vi "SSH_Session.vi"(9 "Processor":i32=2, 11 "Python version":string="3.7") -> (0 "error out":errorcluster, 3 "Python":T1)   [LabVIEW 2019]
uses:
  SerialVIs/PythonCtrl.ctl
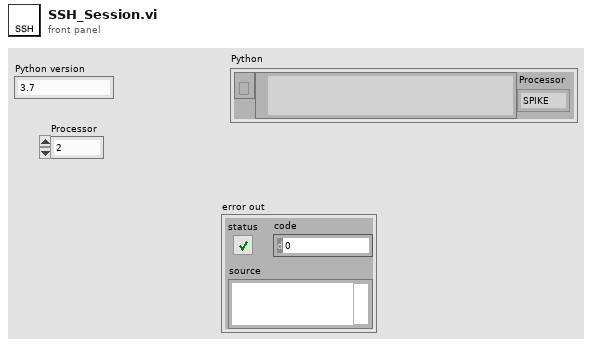
[diagram p1: front panel]
types:
  T1 = typedef "PythonCtrl.ctl" = cluster{"session":refnum<k35>, "PyPath":path, "Processor":enum16{"SPIKE", "Pi", "Pi_ssh"}}
  T2 = cluster{"session out":refnum<k35>, "appended path":path, "Processor":i32}
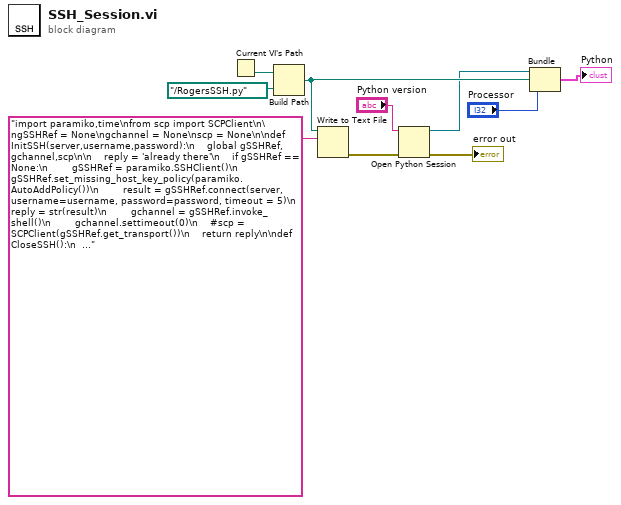
[diagram p0: block diagram]
diagram:
  n1 = Current VI's Path() -> (path=w5:path)
  n2 = Build Path(base path=w5, name or relative path=path "../RogersSSH.py" ("base path")) -> (appended path=w7:path)
  n3 = Write to Text File(file (use dialog)=w7, text="import paramiko,time\nfrom scp import SCPClient\n\ngSSHRef = None\ngchannel = None\nscp = None\n\ndef InitSSH(server,username,password):\n    global gSSHRef, gchannel,scp\n\n    reply = 'already there'\n    if gSSHRef == None:\n        gSSHRef = paramiko.SSHClient()\n        gSSHRef.set_missing_host_key_policy(paramiko.AutoAddPolicy())\n        result = gSSHRef.connect(server, username=username, password=password, timeout = 5)\n        reply = str(result)\n        gchannel = gSSHRef.invoke_shell()\n        gchannel.settimeout(0)\n    #scp = SCPClient(gSSHRef.get_transport())\n    return reply\n\ndef CloseSSH():\n    if gchannel != None:\n        gchannel.close()\n    if gSSHRef != None:\n        gSSHRef.close()\n    if scp != None:\n        scp.close()\n    return('done')\n\ndef WriteSSH(string):\n    global gSSHRef, gchannel,scp\n    reply = 'no reference'\n    if gSSHRef != None:\n        reply = 'no file'\n        if gchannel != None:\n            size = gchannel.send(string.encode())\n            reply = str(size)\n    return reply\n\ndef ReadSSH():\n    global gSSHRef, gchannel,scp\n    reply = 'no reference'\n    if gSSHRef != None:\n        reply = 'no file'\n        if gchannel != None:\n            reply = ''\n            if gchannel.recv_ready():\n                reply = gchannel.recv(9999).decode()\n\n    return(reply)\n\ndef WriteWaitReadSSH(string,char,timeout=10000):\n     global gSSHRef, gchannel,scp\n     reply = ReadSSH()\n     WriteSSH(string)\n     n = int(timeout/10)\n     for i in range(n):\n         ans = ReadSSH()\n         reply = reply + ans\n         if ans.find(char) >= 0:\n             #print(ans)\n             return reply\n         time.sleep(0.01)\n     return reply\n\ndef scp_get(name):\n     try:\n          scp.get(name)\n          return 'get succeeded\\n'\n     except Exception as e:\n          return  'scp.get('+name+')\\n' +str(e)\n\ndef scp_put(source, dest):\n     try:\n          scp.put(source, dest)\n          return 'scp.put('+source+','+dest+')\\n' +'put succeeded\\n'\n     except Exception as e:\n          return str(e)\n\ndef scp_put_all(source, dest):\n     try:\n          scp.put(source, recursive = True, remote_path = dest)\n          return 'put succeeded\\n'\n     except Exception as e:\n          return str(e)\n" ("name or relative path")) -> (error out=w10:errorcluster)  [unwired: 2 in, 2 out]
  n4 = Open Python Session(python version="Python version", 3:w10) -> (session out=w2:refnum<k35>, error out=→"error out":errorcluster)  [unwired: 1 in]
  n5 = Bundle("session out"=w2, "appended path"=w7, "Processor"="Processor") -> (→"Python":T2)  [unwired: 1 in]
